vi "Combined Algorithm.vi"() -> ()   [LabVIEW 2020]
uses:
  <vilib>/MakerHub/LINX/Private/Type Defs/Peripherals/SPI/SPI Configuration.ctl
  <vilib>/MakerHub/LINX/Private/Type Defs/Peripherals/SPI/SPI Bit Order.ctl
  <vilib>/MakerHub/LINX/Private/Type Defs/Peripherals/SPI/SPI Mode.ctl
  <vilib>/MakerHub/LINX/Public/Peripherals/SPI/SPI CS Config.ctl
  <vilib>/MakerHub/LINX/Private/Type Defs/Peripherals/SPI/SPI CS Logic Level.ctl
  <vilib>/MakerHub/LINX/Public/Peripherals/Analog/Analog Read 1 Chan.vi
  <vilib>/MakerHub/LINX/Public/Peripherals/Digital/Digital Write 1 Chan.vi
  <vilib>/MakerHub/LINX/Public/Peripherals/SPI/SPI Write Read 1 Frame.vi
  <vilib>/MakerHub/LINX/Public/Peripherals/PWM/PWM Set Duty Cycle 1 Chan.vi
  <vilib>/MakerHub/LINX/Public/Peripherals/Analog/Analog Read N Chans.vi
  <vilib>/MakerHub/LINX/Public/Peripherals/Digital/Digital Write N Chans.vi
  <vilib>/MakerHub/LINX/Public/Peripherals/SPI/SPI Write Read N Frames.vi
  <vilib>/MakerHub/LINX/Private/Local IO/LinxAnalogRead.vi
  <vilib>/MakerHub/LINX/Public/Utilities/Check Channel.vi
  <vilib>/MakerHub/LINX/Private/Local IO/LinxDigitalWrite.vi
  <vilib>/MakerHub/LINX/Private/Local IO/LinxSpiWriteRead.vi
  <vilib>/MakerHub/LINX/Public/Utilities/Open Serial.vi
  <vilib>/MakerHub/LINX/Private/Utilties/Generate Error.vi
  <vilib>/MakerHub/LINX/Public/Peripherals/PWM/PWM Set Duty Cycle N Chans.vi
  <vilib>/MakerHub/LINX/LMH-LINX.lvlib
panel:
  out "Low Fire Intensity":bool
  out "High Fire intensity":bool
  out "Smoke Sensor Output":dbl(graph)
  out "IR Sensor Output":dbl(graph)
  in  "stop 2":bool
  out "IR Sensor output":dbl
  out "Smoke sensor output Voltage":dbl
  out "Temperature (Celcius)":dbl
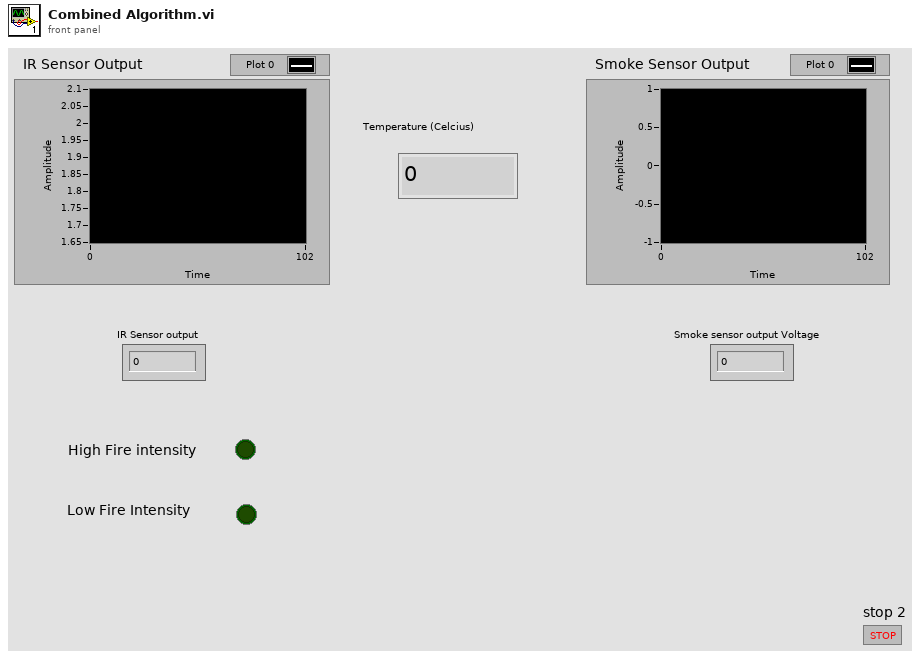
[diagram p1: front panel]
types:
  T1 = typedef "LMH-LINX.lvlib/SPI Configuration.ctl" = cluster{"Clock Frequency":u32, "Bit Order":T2, "SPI Mode":T3}
  T2 = typedef "LMH-LINX.lvlib/SPI Bit Order.ctl" = enum8{"LSb First", "MSb First"}
  T3 = typedef "LMH-LINX.lvlib/SPI Mode.ctl" = enum8{"Mode 0", "Mode 1", "Mode 2", "Mode 3"}
  T4 = typedef "LMH-LINX.lvlib/LINX Ref.ctl" = cluster{"IO":T5, "Interface":T6, "LINX Device Config":T7}
  T5 = typedef "LMH-LINX.lvlib/Platform.ctl" = enum16{"Remote", "Local"}
  T6 = typedef "LMH-LINX.lvlib/Interface.ctl" = enum16{"Serial", "TCP"}
  T7 = typedef "LMH-LINX.lvlib/Device.lvlib/LINX Device Config.ctl" = cluster{"Interface":T6, "COM Port":refnum<visa-resource-name>, "TCP Configuration":T8, "Device Family":u8, "Device ID":u8, "Device Name":string, "TCP Ref":refnum<k5>, "Channels":T9}
  T8 = typedef "LMH-LINX.lvlib/Device.lvlib/TCP Config.ctl" = cluster{"IP Address":string, "Port":u16}
  T9 = typedef "LMH-LINX.lvlib/Channels.ctl" = cluster{"DI":u8[], "DO":u8[], "AI":u8[], "AO":u8[], "PWM":u8[], "QE":u8[], "UART":u8[], "I2C 2":u8[], "SPI":u8[], "CAN":u8[], "Servo":u8[], "AI Ref (V)":dbl, "AI Resolution (Bits)":u8, "AO Ref (V)":dbl, "AO Resolution (Bits)":u8}
  T10 = typedef "LMH-LINX.lvlib/SPI CS Config.ctl" = cluster{"CS Channel":u8, "CS Logic Level":T11}
  T11 = typedef "LMH-LINX.lvlib/SPI CS Logic Level.ctl" = enum8{"Active Low", "Active High"}
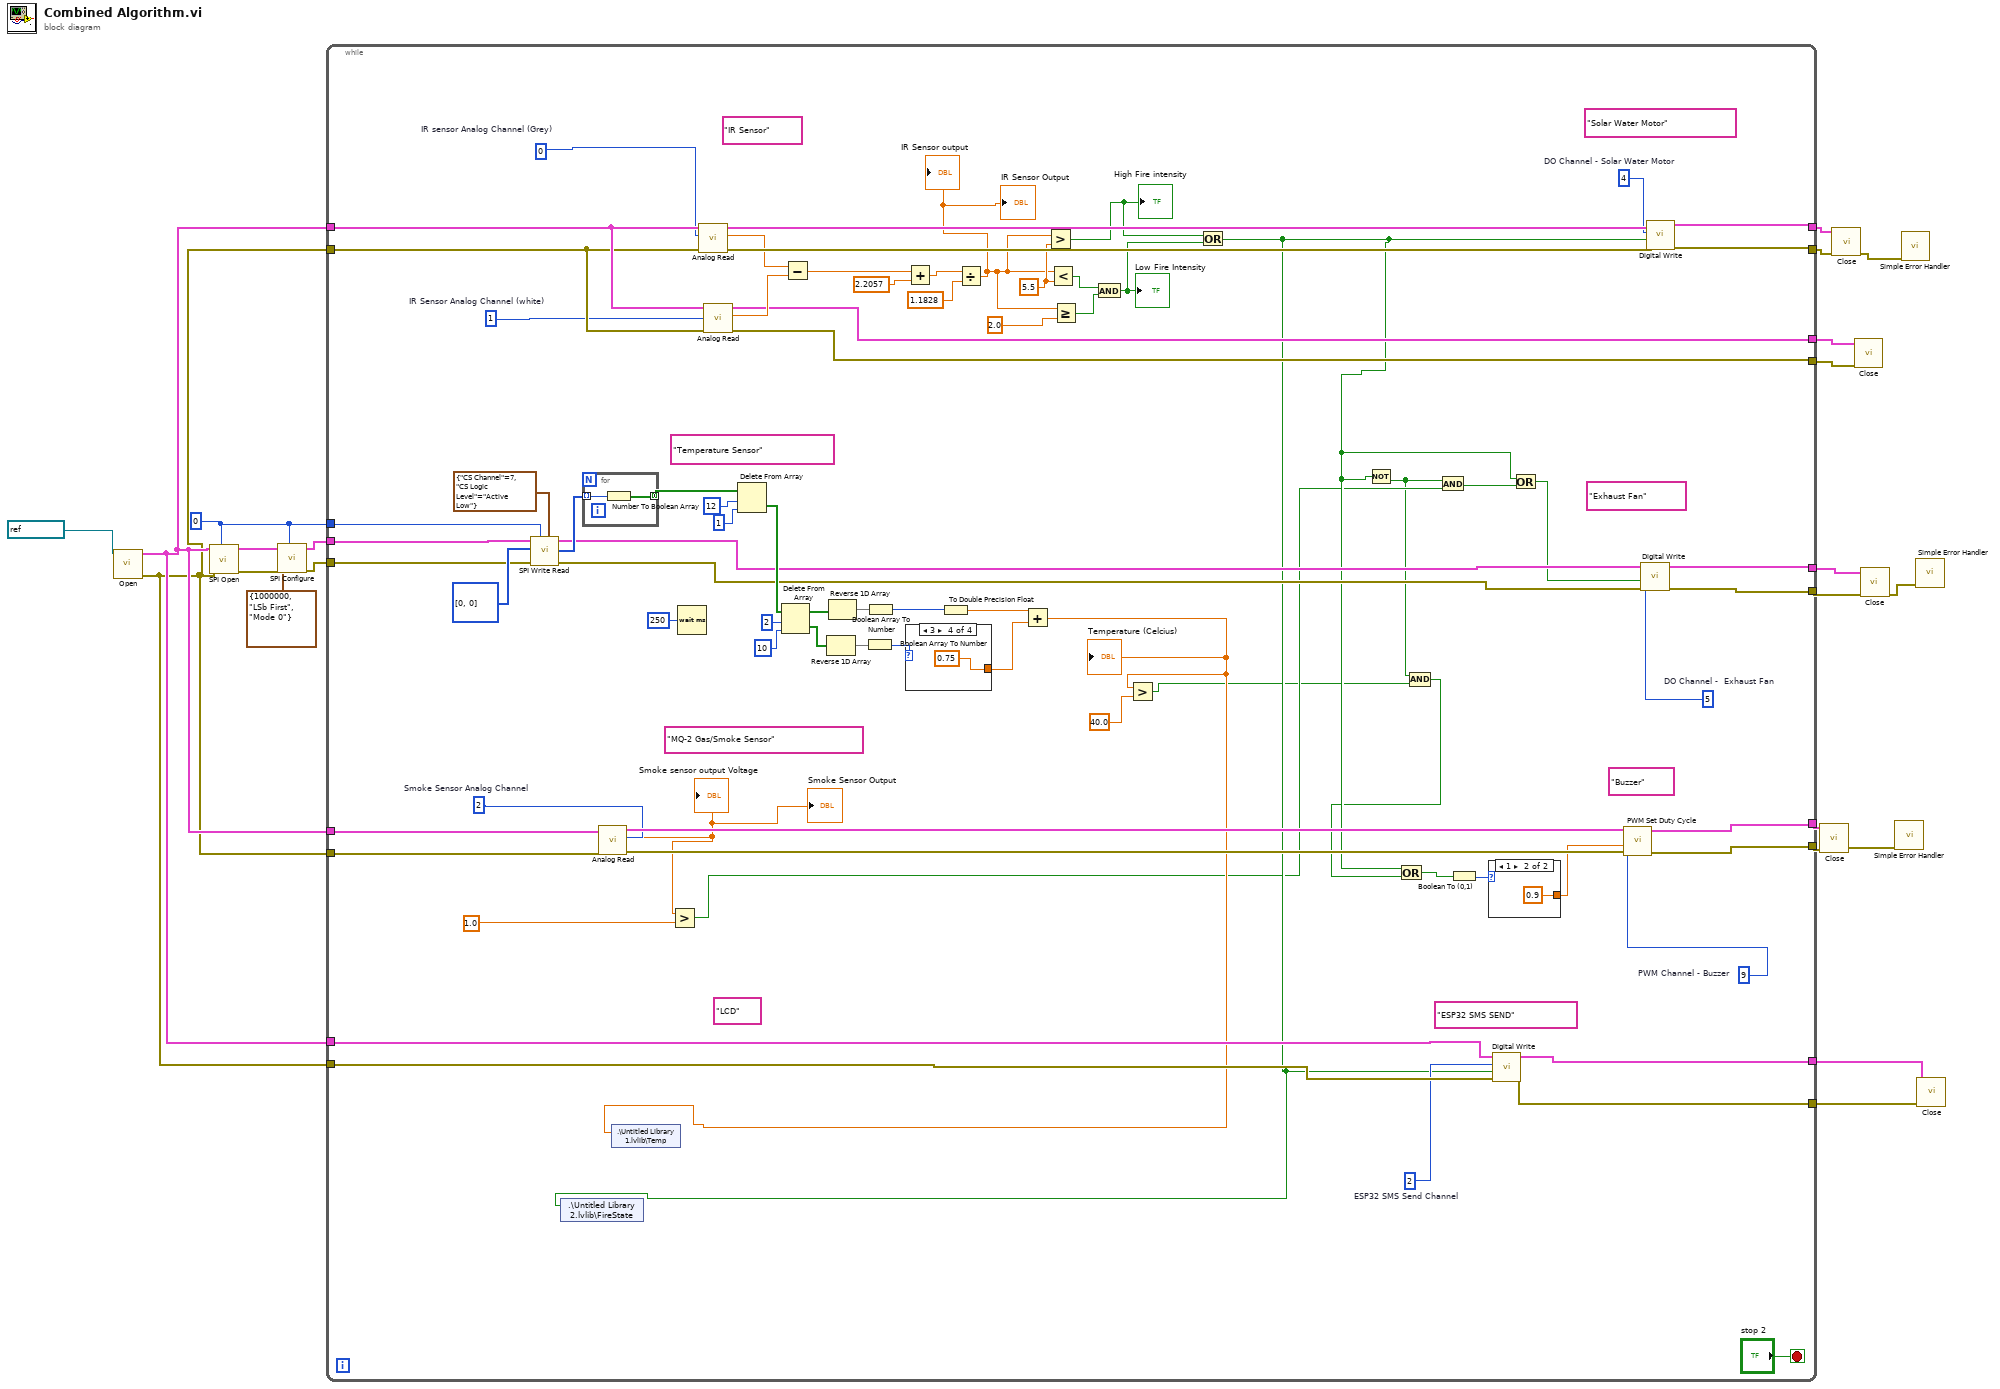
[diagram p0: block diagram]
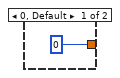
[diagram p2: hidden frame]
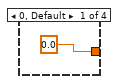
[diagram p3: hidden frame]
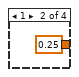
[diagram p4: hidden frame]
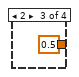
[diagram p5: hidden frame]
diagram:
  w16 = u8 0 ("SPI Channel (0)")
  n1 = call-poly <vilib>:"Open.vi"("Serial Port"=refnum<visa-resource-name> "COM3") -> ("Error Out"=w3:errorcluster, "LINX Resource"=w4:T4)  [unwired: 8 in, 1 out]
  n2 = call <vilib>:"SPI Open.vi"("SPI Channel (0)"=w16, "Error In"=w3, "LINX Resource"=w4) -> ("Error Out"=w21:errorcluster, "LINX Resource"=w20:T4)  [unwired: 7 in]
  n3 = call <vilib>:"SPI Configure.vi"("SPI Channel (0)"=w16, "Error In"=w21, "SPI Configuration"=T1 {"Clock Frequency"=1000000, "Bit Order"=enum."LSb First", "SPI Mode"=enum."Mode 0"}, "LINX Resource"=w20) -> ("Error Out"=w18:errorcluster, "LINX Resource"=w19:T4)  [unwired: 5 in, 1 out]
  n4 = while {
    tunnel: w19 -> [w99]
    tunnel: [w66] -> w10
    tunnel: w18 -> [w82]
    tunnel: [w65] -> w17
    tunnel: w16 -> [w81]
    tunnel: w4 -> [w76]
    tunnel: w3 -> [w75]
    tunnel: [w74] -> w14
    tunnel: [w73] -> w13
    tunnel: w4 -> [w61]
    tunnel: w3 -> [w60]
    tunnel: [w70] -> w12
    tunnel: [w69] -> w11
    tunnel: [w57] -> w6
    tunnel: [w56] -> w5
    tunnel: w4 -> [w51]
    tunnel: w3 -> [w50]
    tunnel: [w53] -> w2
    tunnel: [w54] -> w1
    stop <- "stop 2" stop-if-true
    w37 = 5.5 ("y")
    w43 = u8 9  # PWM Channel - Buzzer
    w44 = u8 5  # DO Channel -  Exhaust Fan
    w45 = u8 4  # DO Channel - Solar Water Motor
    w46 = u8 2  # ESP32 SMS Send Channel
    w47 = u8 2  # Smoke Sensor Analog Channel
    w48 = u8 1  # IR Sensor Analog Channel (white)
    w49 = u8 0  # IR sensor Analog Channel (Grey)
    (unwired) "ESP32 SMS SEND"
    (unwired) "LCD"
    (unwired) "Exhaust Fan"
    (unwired) "Buzzer"
    (unwired) "Solar Water Motor"
    (unwired) "IR Sensor"
    (unwired) "Temperature Sensor"
    (unwired) "MQ-2 Gas/Smoke Sensor"
    n5 = call-poly <vilib>:"SPI Write Read.vi"("CS Configuration"=T10 {"CS Channel"=7, "CS Logic Level"=enum."Active Low"}, "SPI Channel (0)"=w81, "Error In"=w82, "Data"=u16[] [0, 0], "LINX Resource"=w99) -> ("Error Out"=w67:errorcluster, "Read Data"=w97:u8[], "LINX Resource"=w68:T4)  [unwired: 4 in]
    n6 = for {
      tunnel: w97 -> [w108] mode=indexing
      tunnel: [w107] -> w80 mode=concatenating
      n7 = Number To Boolean Array(number=w108) -> (Boolean array=w107:bool[])
    }
    n8 = call-poly <vilib>:"Analog Read.vi"("Error In"=w75, "Analog Channel"=w47, "LINX Resource"=w76) -> ("Error Out"=w78:errorcluster, "Voltage"=w42:dbl, "LINX Resource"=w79:T4)  [unwired: 5 in, 1 out]
    "Smoke sensor output Voltage" <- w42
    "Smoke Sensor Output" <- w42
    n9 = Greater?(x=w42, y=1.0) -> (0:w26:bool)
    n10 = Wait (ms)(milliseconds to wait=u32 250) -> ()  [unwired: 1 out]
    n11 = call-poly <vilib>:"Analog Read.vi"("Error In"=w60, "Analog Channel"=w49, "LINX Resource"=w61) -> ("Error Out"=w71:errorcluster, "Voltage"=w59:dbl, "LINX Resource"=w72:T4)  [unwired: 5 in, 1 out]
    n12 = call-poly <vilib>:"Analog Read.vi"("Error In"=w60, "Analog Channel"=w48, "LINX Resource"=w61) -> ("Error Out"=w56:errorcluster, "Voltage"=w58:dbl, "LINX Resource"=w57:T4)  [unwired: 5 in, 1 out]
    n13 = Delete From Array(array=w80, length=12, index=1) -> (deleted portion=w93:bool[])  [unwired: 1 out]
    n14 = Delete From Array(array=w93, length=2, index=10) -> (deleted portion=w89:bool[], array with subset deleted=w90:bool[])
    n15 = Subtract(x=w59, y=w58) -> (x-y=w41:dbl)
    n16 = Reverse 1D Array(array=w89) -> (reversed array=w87:bool[])
    n17 = Reverse 1D Array(array=w90) -> (reversed array=w88:bool[])
    n18 = Boolean Array To Number(Boolean array=w87) -> (number=w86:u32)
    n19 = Boolean Array To Number(Boolean array=w88) -> (number=w83:u32)
    n20 = Add(x=w41, y=2.2057) -> (x+y=w39:dbl)
    n21 = case shown="3" w86 {
      tunnel: [0.0 0.25 0.5 0.75] -> w85
      frame 0, Default {
      }
      frame 1 {
      }
      frame 2 {
      }
      frame 3 {
      }
    }
    n22 = To Double Precision Float(number=w83) -> (double precision float=w84:dbl)
    n23 = Divide(x=w39, y=1.1828) -> (x/y=w36:dbl)
    "IR Sensor output" <- w36
    "IR Sensor Output" <- w36
    n24 = Add(x=w84, y=w85) -> (x+y=w30:dbl)
    "Temperature (Celcius)" <- w30
    n25 = shared-variable ".\\Untitled Library 1.lvlib\\Temp"(w30) -> ()  [unwired: 1 in, 1 out]
    n26 = Greater?(x=w36, y=w37) -> (0:w32:bool)
    "High Fire intensity" <- w32
    n27 = Less?(x=w36, y=w37) -> (x < y?=w34:bool)
    n28 = Greater Or Equal?(x=w36, y=2.0) -> (x >= y?=w33:bool)
    n29 = And(x=w34, y=w33) -> (x .and. y?=w31:bool)
    "Low Fire Intensity" <- w31
    n30 = Greater?(x=w30, y=40.0) -> (0:w24:bool)
    n31 = Or(x=w32, y=w31) -> (x .or. y?=w29:bool)
    n32 = shared-variable ".\\Untitled Library 2.lvlib\\FireState"(w29) -> ()  [unwired: 1 in, 1 out]
    n33 = Not(x=w29) -> (.not. x?=w25:bool)
    n34 = And(x=w25, y=w24) -> (x .and. y?=w23:bool)
    n35 = Or(x=w29, y=w23) -> (x .or. y?=w62:bool)
    n36 = And(x=w25, y=w26) -> (x .and. y?=w27:bool)
    n37 = Boolean To (0,1)(Boolean=w62) -> (0, 1=w77:i16)
    n38 = case shown="1" w77 {
      tunnel: [0 0.9] -> w63
      frame 0, Default {
      }
      frame 1 {
      }
    }
    n39 = call-poly <vilib>:"Digital Write.vi"("Error In"=w50, "Output Value"=w29, "DO Channel"=w46, "LINX Resource"=w51) -> ("Error Out"=w53:errorcluster, "LINX Resource"=w54:T4)  [unwired: 6 in]
    n40 = Or(x=w29, y=w27) -> (x .or. y?=w55:bool)
    n41 = call-poly <vilib>:"PWM Set Duty Cycle.vi"("Error In"=w78, "Duty Cycle (0-1)"=w63, "PWM Channel"=w43, "LINX Resource"=w79) -> ("Error Out"=w73:errorcluster, "LINX Resource"=w74:T4)  [unwired: 6 in]
    n42 = call-poly <vilib>:"Digital Write.vi"("Error In"=w67, "Output Value"=w55, "DO Channel"=w44, "LINX Resource"=w68) -> ("Error Out"=w65:errorcluster, "LINX Resource"=w66:T4)  [unwired: 6 in]
    n43 = call-poly <vilib>:"Digital Write.vi"("Error In"=w71, "Output Value"=w29, "DO Channel"=w45, "LINX Resource"=w72) -> ("Error Out"=w69:errorcluster, "LINX Resource"=w70:T4)  [unwired: 6 in]
  }
  n44 = call <vilib>:"Close.vi"("Error In"=w13, "LINX Resource"=w14) -> ("Error Out"=w9:errorcluster)  [unwired: 9 in]
  n45 = call <vilib>:"Close.vi"("Error In"=w11, "LINX Resource"=w12) -> ("Error Out"=w7:errorcluster)  [unwired: 9 in]
  n46 = call <vilib>:"Close.vi"("Error In"=w5, "LINX Resource"=w6) -> ()  [unwired: 9 in, 1 out]
  n47 = call <vilib>:"Close.vi"("Error In"=w17, "LINX Resource"=w10) -> ("Error Out"=w8:errorcluster)  [unwired: 9 in]
  n48 = call <vilib>:"Simple Error Handler.vi"("error in (no error)"=w9) -> ()  [unwired: 4 in, 5 out]
  n49 = call <vilib>:"Simple Error Handler.vi"("error in (no error)"=w7) -> ()  [unwired: 4 in, 5 out]
  n50 = call <vilib>:"Simple Error Handler.vi"("error in (no error)"=w8) -> ()  [unwired: 4 in, 5 out]
  n51 = call <vilib>:"Close.vi"("Error In"=w2, "LINX Resource"=w1) -> ()  [unwired: 9 in, 1 out]
